vi "vision processing.vi"(6 "Image In":T1, 7 "error in (no error)":errorcluster) -> (11 "error out":errorcluster, 14 "x":dbl, 15 "y":dbl, 16 "left":dbl, 17 "top":dbl, 18 "right":dbl, 19 "bottom":dbl)   [LabVIEW 2012]
uses:
  <vilib>/vision/Image Controls.llb/IMAQ Image.ctl
  typedefs/fg_typedef.ctl
  <vilib>/vision/NI_Vision_Development_Module.lvlib
panel:
  out "Cam":T1(plugin-control)
  out "# Particles":i32
  in  "error in":errorcluster
  out "Image Out":T1
  out "error out":errorcluster
  out "Number of Particles Found":i32
  out "Image Out":T1(plugin-control)
  out "Number of Targets Found":i32
  # "0  center of mass x\n1  center of mass y\n2  first pixel x\n3  first pixel y\n4  bounding rect left\n5  bounding rect top\n6  bounding rect right\n7  bounding rect bottom\n8 max feret diameter start x\n9  max feret diameter start y\n10 max feret diameter end x\n11 max feret diameter end y\n12 max horiz segment length left\n13 max horiz segment length right\n14 max horiz segment length row\n15 bounding rect width \n16 bounding rect height\n17 bounding rect diagional\n..\n33 area"
  # "13'3\"\n3'9\""
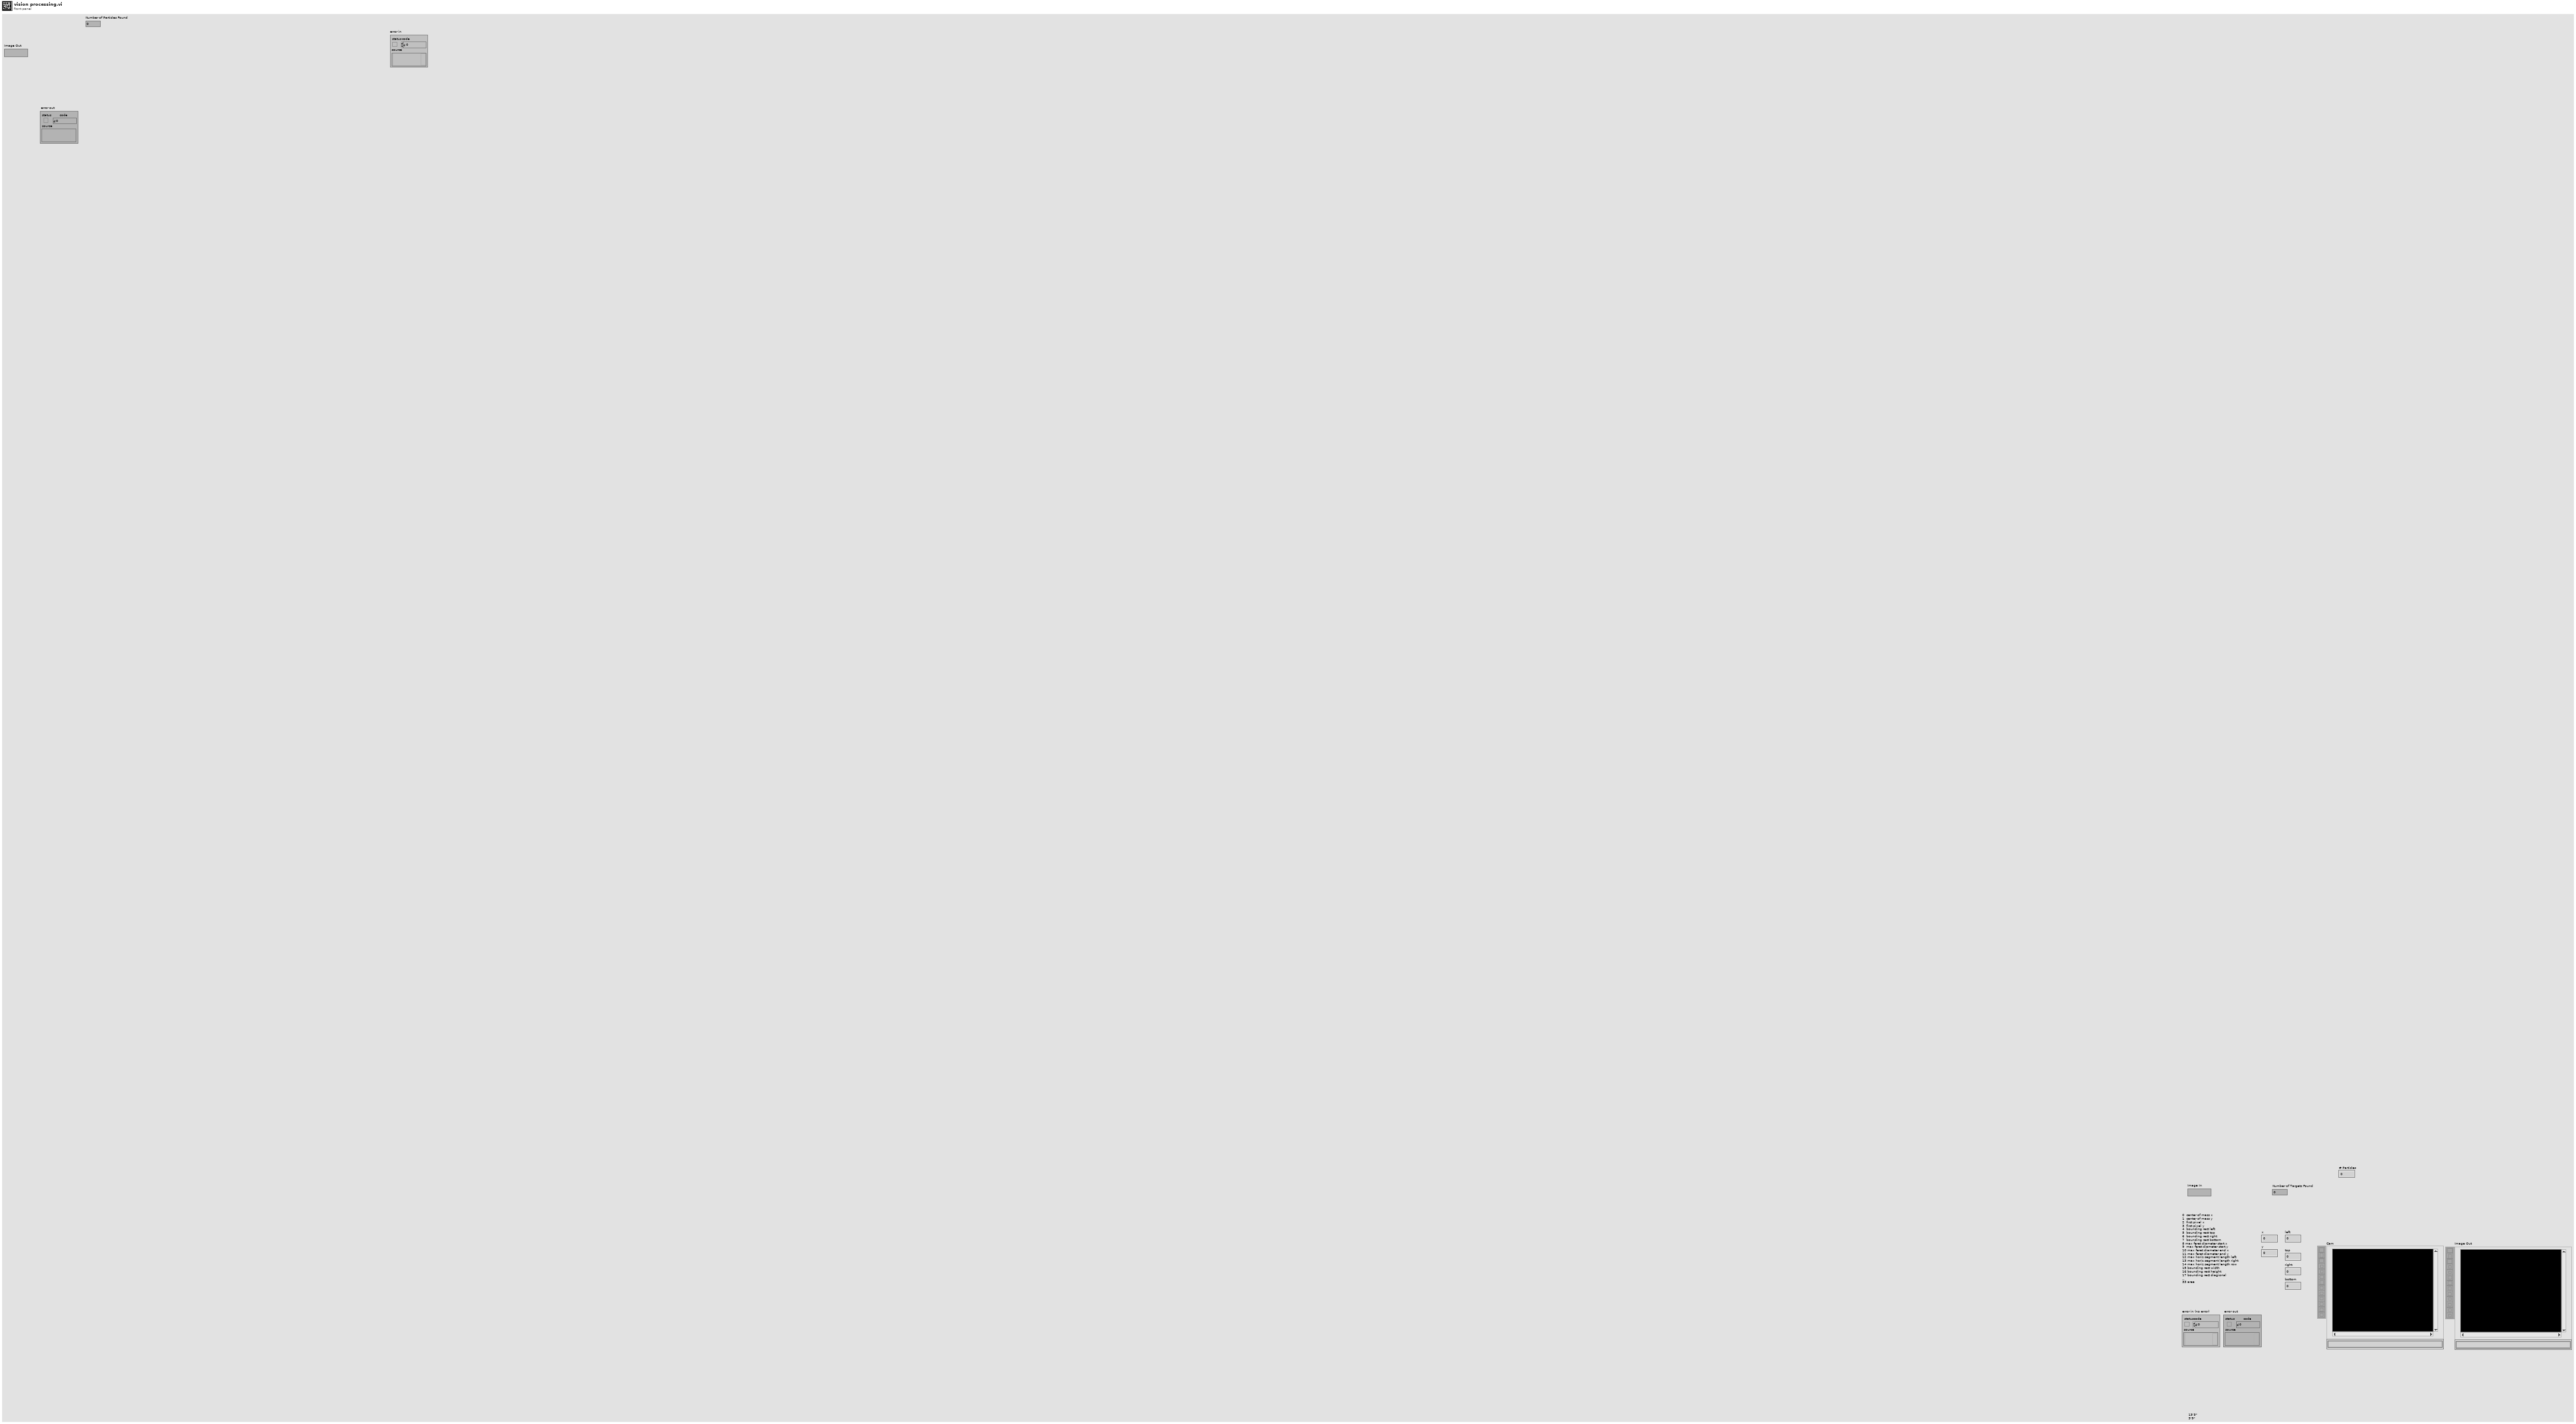
[diagram p1: front panel]
types:
  T1 = typedef "IMAQ Image.ctl" = refnum<image>
  T2 = typedef "Image Type" = u32
  T3 = typedef "fg_typedef.ctl" = enum16{"Get", "Set"}
  T4 = enum32{"AutoM", "Close", "Dilate", "Erode", "Gradient", "Gradient out", "Gradient in", "Hit miss", "Open", "PClose", "POpen", "Thick", "Thin"}
  T5 = cluster{"Brightness":sgl, "Contrast":sgl, "Gamma":sgl}
  T6 = cluster{"Measurement Parameter":i32, "Range Lower Value":dbl, "Range Upper Value":dbl, "Range":bool, "Measurement Type":bool}[]
  T7 = typedef "Particle Parameters" = i32
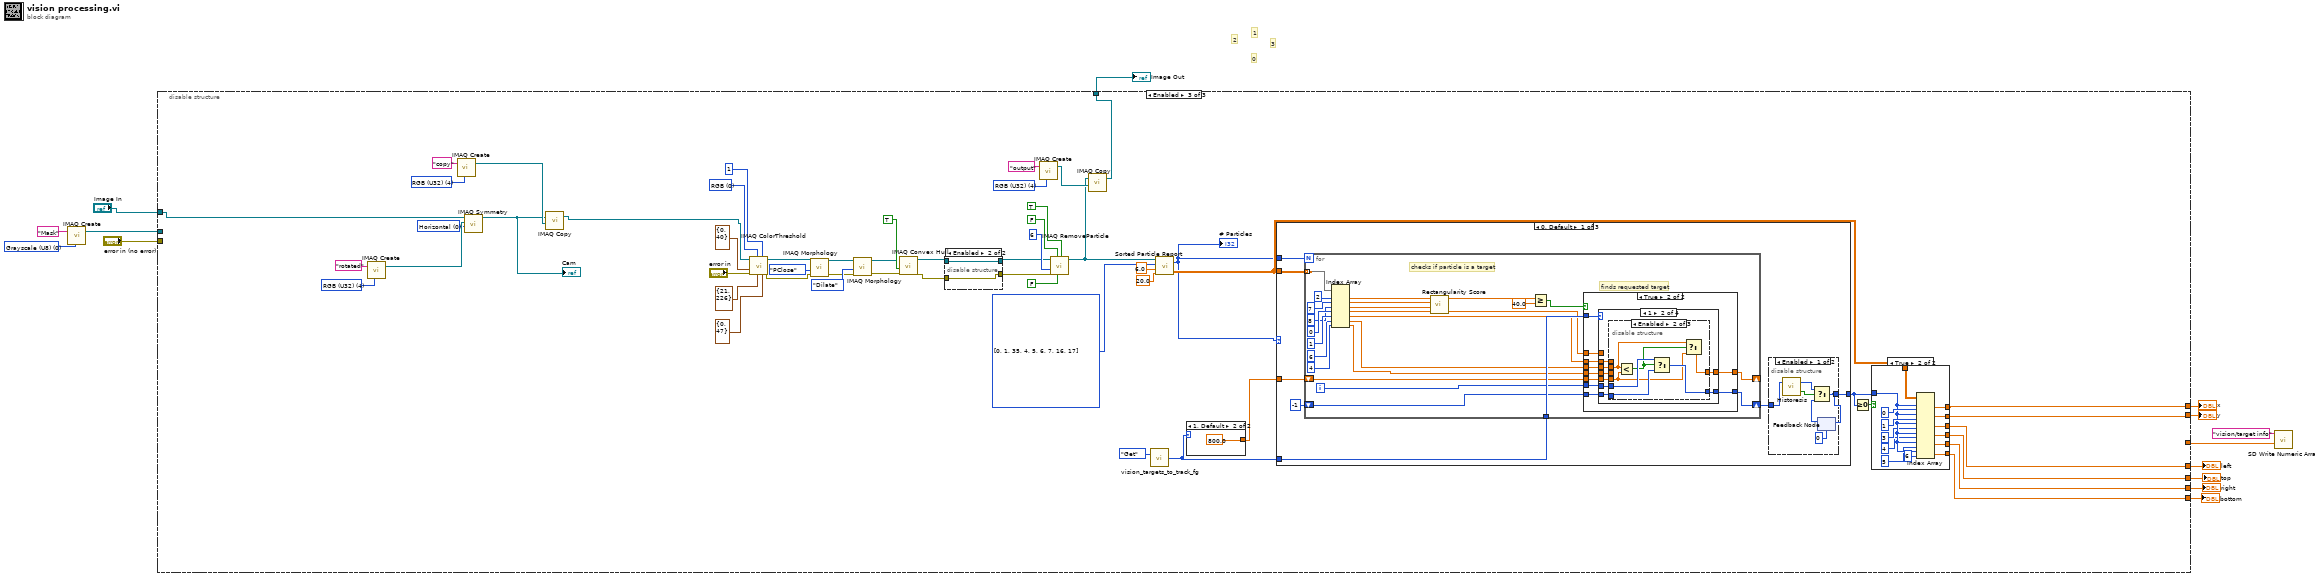
[diagram p0: block diagram]
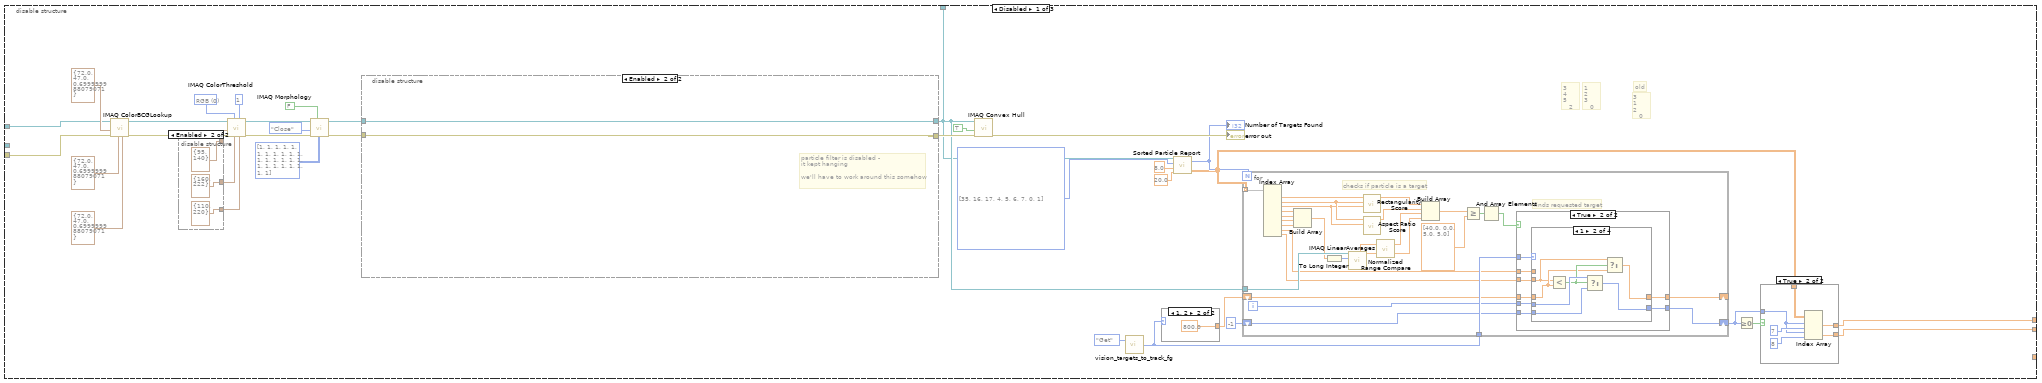
[diagram p2: hidden frame]
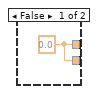
[diagram p3: hidden frame]
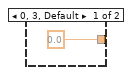
[diagram p4: hidden frame]
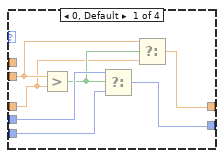
[diagram p6: hidden frame]
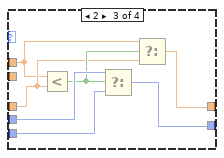
[diagram p7: hidden frame]
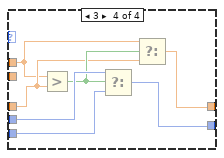
[diagram p8: hidden frame]
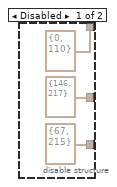
[diagram p9: hidden frame]
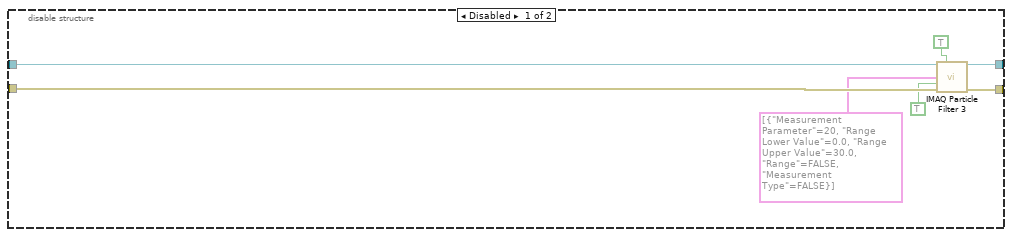
[diagram p10: hidden frame]
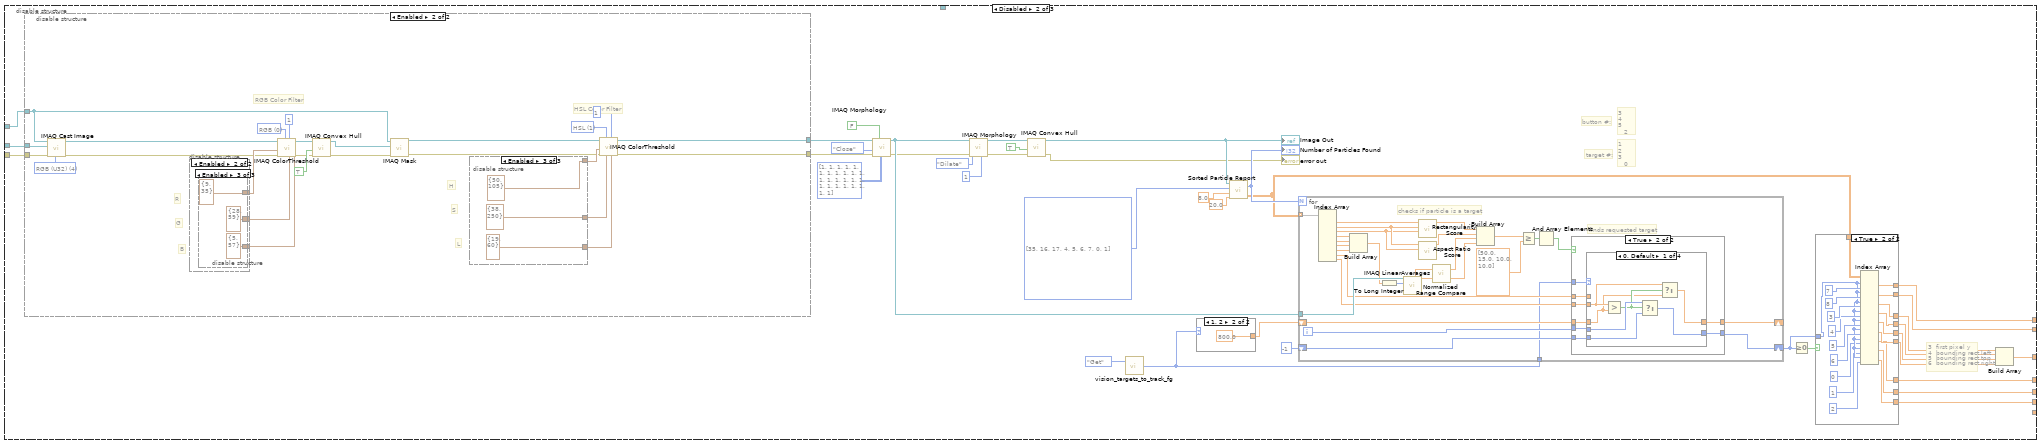
[diagram p11: hidden frame]
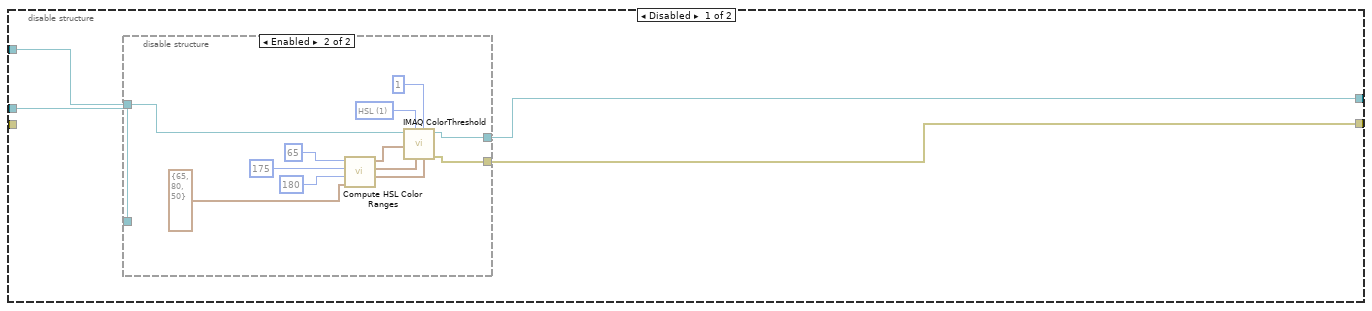
[diagram p12: hidden frame]
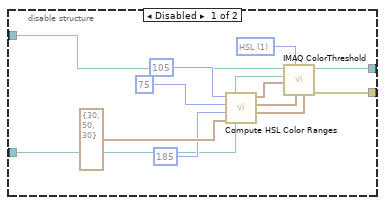
[diagram p13: hidden frame]
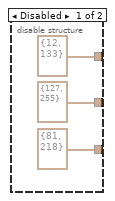
[diagram p14: hidden frame]
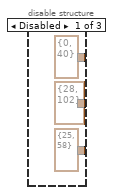
[diagram p15: hidden frame]
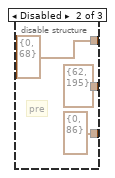
[diagram p16: hidden frame]
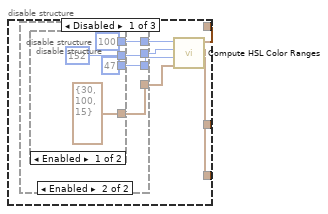
[diagram p17: hidden frame]
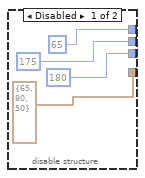
[diagram p18: hidden frame]
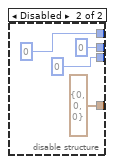
[diagram p19: hidden frame]
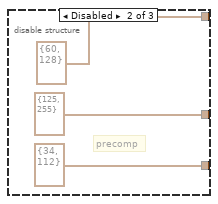
[diagram p20: hidden frame]
diagram:
  w11 = T2 0 items=["Grayscale (U8)", "Grayscale (I16)", "Grayscale (SGL)", "Complex (CSG)", "RGB (U32)", "HSL (U32)", "RGB (U64)", "Grayscale (U16)"] ("Image Type")
  # "3"
  # "2"
  # "1"
  # "0"
  n1 = call "IMAQ Create"("Image Name"="Mask", "Image Type"=w11) -> ("New Image"=w10:T1)  [unwired: 2 in, 2 out]
  n2 = disable-structure shown="Enabled" {
    disable-tunnel: "error in (no error)" -> [w32 w154 _]
    disable-tunnel: "Image In" -> [w31 w166 w372]
    disable-tunnel: [w17 w163 w384] -> w9
    disable-tunnel: [w16 w144 w373] -> w8
    disable-tunnel: w10 -> [_ w155 _]
    disable-tunnel: [_ w153 w383] -> w7
    disable-tunnel: [_ w152 w374] -> w6
    disable-tunnel: [_ w151 w382] -> w5
    disable-tunnel: [_ w143 _] -> w4
    disable-tunnel: [w15 _ w391] -> w2
    disable-tunnel: [_ _ w375] -> w1
    frame Disabled {
      w24 = T7[] [35, 16, 17, 4, 5, 6, 7, 0, 1] items=["Center of Mass X", "Center of Mass Y", "First Pixel X", "First Pixel Y", "Bounding Rect Left", "Bounding Rect Top", "Bounding Rect Right", "Bounding Rect Bottom", "Max Feret Diameter Start X", "Max Feret Diameter Start Y", "Max Feret Diameter End X", "Max Feret Diameter End Y", "Max Horiz. Segment Length Left", "Max Horiz. Segment Length Right", "Max Horiz. Segment Length Row", "-", "Bounding Rect Width", "Bounding Rect Height", "Bounding Rect Diagonal", "Perimeter", "Convex Hull Perimeter", "Holes' Perimeter", "Max Feret Diameter", "Equivalent Ellipse Major Axis", "Equivalent Ellipse Minor Axis", "Equivalent Ellipse Minor Axis (Feret)", "Equivalent Rect Long Side", "Equivalent Rect Short Side", "Equivalent Rect Diagonal", "Equivalent Rect Short Side (Feret)", "Average Horiz. Segment Length", "Average Vert. Segment Length", "Hydraulic Radius", "Waddel Disk Diameter", "-", "Area", "Holes' Area", "Particle & Holes' Area", "Convex Hull Area", "Image Area", "-", "Number of Holes", "Number of Horiz. Segments", "Number of Vert. Segments", "-", "Orientation", "Max Feret Diameter Orientation", "-", "% Area/Image Area", "% Area/(Particle & Holes' Area)", "Ratio of Equivalent Ellipse Axes", "Ratio of Equivalent Rect Sides", "-", "Elongation Factor", "Compactness Factor", "Heywood Circularity Factor", "Type Factor", "-", "Sum X", "Sum Y", "Sum XX", "Sum XY", "Sum YY", "Sum XXX", "Sum XXY", "Sum XYY", "Sum YYY", "-", "Moment of Inertia XX", "Moment of Inertia XY", "Moment of Inertia YY", "Moment of Inertia XXX", "Moment of Inertia XXY", "Moment of Inertia XYY", "Moment of Inertia YYY", "Norm. Moment of Inertia XX", "Norm. Moment of Inertia XY", "Norm. Moment of Inertia YY", "Norm. Moment of Inertia XXX", "Norm. Moment of Inertia XXY", "Norm. Moment of Inertia XYY", "Norm. Moment of Inertia YYY", "Hu Moment 1", "Hu Moment 2", "Hu Moment 3", "Hu Moment 4", "Hu Moment 5", "Hu Moment 6", "Hu Moment 7"] ("Requested Particle Measurements")
      w46 = u16 0 items=["RGB", "HSL", "HSV", "HSI"] ("Color Mode")
      # "old"
      # "1   \n2     3\n   0"
      # "3   \n1     2\n   0"
      # "3   \n4     5\n   2"
      n3 = call "IMAQ ColorBCGLookup"("Blue BCG Values"=T5 {"Brightness"=72.0, "Contrast"=47.0, "Gamma"=0.7}, "Green BCG Values"=T5 {"Brightness"=72.0, "Contrast"=47.0, "Gamma"=0.7}, "error in (no error)"=w32, "Red BCG Values"=T5 {"Brightness"=72.0, "Contrast"=47.0, "Gamma"=0.7}, "Image Src"=w31) -> ("error out"=w51:errorcluster, "Image Dst Out"=w42:T1)  [unwired: 2 in, 3 out]
      n4 = disable-structure shown="Enabled" {
        disable-tunnel: [cluster{"Lower value":i32, "Upper value":i32} {"Lower value"=0, "Upper value"=110} ("Red or Hue Range") cluster{"Lower value":i32, "Upper value":i32} {"Lower value"=95, "Upper value"=140} ("Red or Hue Range")] -> w45
        disable-tunnel: [cluster{"Lower value":i32, "Upper value":i32} {"Lower value"=146, "Upper value"=217} ("Green or Sat Range") cluster{"Lower value":i32, "Upper value":i32} {"Lower value"=160, "Upper value"=222} ("Green or Sat Range")] -> w44
        disable-tunnel: [cluster{"Lower value":i32, "Upper value":i32} {"Lower value"=67, "Upper value"=215} ("Blue or Luma or Val or Inten Range") cluster{"Lower value":i32, "Upper value":i32} {"Lower value"=110, "Upper value"=220} ("Blue or Luma or Val or Inten Range")] -> w43
        frame Disabled {
        }
        frame Enabled {
        }
      }
      n5 = call "IMAQ ColorThreshold"("Blue or Luma or Val or Inten Range"=w43, "Replace Value"=1, "Green or Sat Range"=w44, "Color Mode"=w46, "error in (no error)"=w51, "Red or Hue Range"=w45, "Image Src"=w42) -> ("error out"=w41:errorcluster, "Image Dst Out"=w37:T1)  [unwired: 1 in, 2 out]
      n6 = call "IMAQ Morphology"("Structuring Element"=i32[][] [[1, 1, 1, 1, 1], [1, 1, 1, 1, 1], [1, 1, 1, 1, 1], [1, 1, 1, 1, 1], [1, 1, 1, 1, 1]], "Square/Hexa (Square)"=FALSE, "error in (no error)"=w41, "Operation"=T4."Close", "Image Src"=w37) -> ("error out"=w36:errorcluster, "Image Dst Out"=w34:T1)  [unwired: 2 in, 3 out]
      n7 = disable-structure shown="Enabled" {
        disable-tunnel: w36 -> [w140 w142]
        disable-tunnel: [w137 w142] -> w35
        disable-tunnel: w34 -> [w136 w141]
        disable-tunnel: [w134 w141] -> w30
        frame Disabled {
          n8 = call "IMAQ Particle Filter 3"("Image Src"=w136, "Connectivity 4/8 (8)"=TRUE, "Selection Values"=T6 [{"Measurement Parameter"=20, "Range Lower Value"=0.0, "Range Upper Value"=30.0, "Range"=FALSE, "Measurement Type"=FALSE}], "Keep/Remove Particles (F)"=TRUE ("Keep/Remove Particles"), "error in (no error)"=w140) -> ("Image Dst Out"=w134:T1, "error out"=w137:errorcluster)  [unwired: 4 in, 5 out]
        }
        frame Enabled {
          # "particle filter is disabled - \nit kept hanging\n\nwe'll have to work around this somehow"
        }
      }
      n9 = call "IMAQ Convex Hull"("error in (no error)"=w35, "Connectivity 4/8 (8)"=TRUE, "Image Src"=w30) -> ("error out"=→"error out":errorcluster, "Image Dst Out"=w15:T1)  [unwired: 1 in, 6 out]
      n10 = call "vision_targets_to_track_fg.vi"("Menu (Get)"=fg_typedef."Get") -> ("Output"=w27:i32)  [unwired: 1 in]
      n11 = case shown="1, 2" w27 {
        tunnel: [0.0 ("element") 800.0 ("element")] -> w28
        frame 0, 3, Default {
        }
        frame 1, 2 {
        }
      }
      n12 = call "Sorted Particle Report.vi"("Area Size Limit"=20.0, "Particle Count Limit"=8.0, "Pixel Measurements"=w24, "Image in"=w15) -> ("Sorted Data"=w20:dbl[][], "Particles"=w21:i32)
      "Number of Targets Found" <- w21
      n13 = for {
        N: w21 -> [_]
        tunnel: w30 -> [w89]
        tunnel: w20 -> [w88] mode=indexing
        tunnel: w27 -> [w78]
        shift-right: [w70] -> _
        shift-left: w28 -> [w73]
        shift-right: [w71] -> w19
        shift-left: -1 -> [w72]
        i -> [w74]
        # "checks if particle is a target"
        # "finds requested target"
        n14 = Index Array(array=w88) -> (element #1=w69:dbl, element #2=w66:dbl, element #3=w65:dbl, element #4=w84:dbl, element #5=w83:dbl, element #6=w82:dbl, element #7=w81:dbl, element #8=w76:dbl, element #9=w77:dbl)  [unwired: 9 in]
        n15 = Build Array(w84, w83, w82, w81) -> (w80:dbl[])
        n16 = To Long Integer(number=w80) -> (32bit integer=w79:i32[])
        n17 = call "IMAQ LinearAverages"("Optional Rectangle"=w79, "Image Src"=w89) -> ("Y Axis Averages"=w61:sgl[], "X Axis Averages"=w62:sgl[])  [unwired: 2 in, 6 out]
        n18 = call "Rectangularity Score.vi"("Height"=w65, "Width"=w66, "Area"=w69) -> ("Score"=w68:dbl)  [unwired: 8 in]
        n19 = call "Aspect Ratio Score.vi"("Height"=w65, "Width"=w66) -> ("Score"=w67:dbl)  [unwired: 9 in]
        n20 = call "Normalized Range Compare.vi"("Y Averages"=w61, "X Averages"=w62) -> ("Y Score"=w63:dbl, "X Score"=w64:dbl)
        n21 = Build Array(w68, w67, w64, w63) -> (w87:dbl[])
        n22 = Greater Or Equal?(x=w87, y=dbl[] [40.0, 0.0, 5.0, 5.0]) -> (x >= y?=w85:bool[])
        n23 = And Array Elements(Boolean array=w85) -> (logical AND=w75:bool)
        n24 = case shown="True" w75 {
          tunnel: w78 -> [_ w99]
          tunnel: w77 -> [_ w98]
          tunnel: w76 -> [_ w97]
          tunnel: w74 -> [_ w96]
          tunnel: w73 -> [w90 w95]
          tunnel: w72 -> [w91 w94]
          tunnel: [w91 w93] -> w71
          tunnel: [w90 w92] -> w70
          frame False {
          }
          frame True {
            n25 = case shown="1" w99 {
              tunnel: w98 -> [w102 w107 _ _]
              tunnel: w97 -> [_ _ w114 w121]
              tunnel: w96 -> [w106 w113 w120 w127]
              tunnel: w95 -> [w101 w109 w116 w123]
              tunnel: w94 -> [w105 w112 w119 w126]
              tunnel: [w104 w111 w118 w125] -> w93
              tunnel: [w100 w108 w115 w122] -> w92
              frame 0, Default {
                n26 = Greater?(x=w102, y=w101) -> (0:w103:bool)
                n27 = Select(t=w106, s=w103, f=w105) -> (s? t:f=w104:i32)
                n28 = Select(t=w102, s=w103, f=w101) -> (s? t:f=w100:dbl)
              }
              frame 1 {
                n29 = Less?(x=w107, y=w109) -> (x < y?=w110:bool)
                n30 = Select(t=w113, s=w110, f=w112) -> (s? t:f=w111:i32)
                n31 = Select(t=w107, s=w110, f=w109) -> (s? t:f=w108:dbl)
              }
              frame 2 {
                n32 = Less?(x=w114, y=w116) -> (x < y?=w117:bool)
                n33 = Select(t=w120, s=w117, f=w119) -> (s? t:f=w118:i32)
                n34 = Select(t=w114, s=w117, f=w116) -> (s? t:f=w115:dbl)
              }
              frame 3 {
                n35 = Greater?(x=w121, y=w123) -> (0:w124:bool)
                n36 = Select(t=w127, s=w124, f=w126) -> (s? t:f=w125:i32)
                n37 = Select(t=w121, s=w124, f=w123) -> (s? t:f=w122:dbl)
              }
            }
          }
        }
      }
      n38 = Greater Or Equal To 0?(x=w19) -> (x >= 0?=w18:bool)
      n39 = case shown="True" w18 {
        tunnel: [w52 w56] -> w17
        tunnel: [w52 w55] -> w16
        tunnel: w20 -> [_ w54]
        tunnel: w19 -> [_ w53]
        frame False {
          w52 = 0.0 ("Numeric")
        }
        frame True {
          n40 = Index Array(array=w54, index (row) #1=w53, index (col) #1=7, index (row) #2=w53, index (col) #2=8) -> (element #1=w56:dbl, element #2=w55:dbl)
        }
      }
    }
    frame Disabled {
      w165 = T7[] [35, 16, 17, 4, 5, 6, 7, 0, 1] items=["Center of Mass X", "Center of Mass Y", "First Pixel X", "First Pixel Y", "Bounding Rect Left", "Bounding Rect Top", "Bounding Rect Right", "Bounding Rect Bottom", "Max Feret Diameter Start X", "Max Feret Diameter Start Y", "Max Feret Diameter End X", "Max Feret Diameter End Y", "Max Horiz. Segment Length Left", "Max Horiz. Segment Length Right", "Max Horiz. Segment Length Row", "-", "Bounding Rect Width", "Bounding Rect Height", "Bounding Rect Diagonal", "Perimeter", "Convex Hull Perimeter", "Holes' Perimeter", "Max Feret Diameter", "Equivalent Ellipse Major Axis", "Equivalent Ellipse Minor Axis", "Equivalent Ellipse Minor Axis (Feret)", "Equivalent Rect Long Side", "Equivalent Rect Short Side", "Equivalent Rect Diagonal", "Equivalent Rect Short Side (Feret)", "Average Horiz. Segment Length", "Average Vert. Segment Length", "Hydraulic Radius", "Waddel Disk Diameter", "-", "Area", "Holes' Area", "Particle & Holes' Area", "Convex Hull Area", "Image Area", "-", "Number of Holes", "Number of Horiz. Segments", "Number of Vert. Segments", "-", "Orientation", "Max Feret Diameter Orientation", "-", "% Area/Image Area", "% Area/(Particle & Holes' Area)", "Ratio of Equivalent Ellipse Axes", "Ratio of Equivalent Rect Sides", "-", "Elongation Factor", "Compactness Factor", "Heywood Circularity Factor", "Type Factor", "-", "Sum X", "Sum Y", "Sum XX", "Sum XY", "Sum YY", "Sum XXX", "Sum XXY", "Sum XYY", "Sum YYY", "-", "Moment of Inertia XX", "Moment of Inertia XY", "Moment of Inertia YY", "Moment of Inertia XXX", "Moment of Inertia XXY", "Moment of Inertia XYY", "Moment of Inertia YYY", "Norm. Moment of Inertia XX", "Norm. Moment of Inertia XY", "Norm. Moment of Inertia YY", "Norm. Moment of Inertia XXX", "Norm. Moment of Inertia XXY", "Norm. Moment of Inertia XYY", "Norm. Moment of Inertia YYY", "Hu Moment 1", "Hu Moment 2", "Hu Moment 3", "Hu Moment 4", "Hu Moment 5", "Hu Moment 6", "Hu Moment 7"] ("Requested Particle Measurements")
      # "3  first pixel y\n4  bounding rect left\n5  bounding rect top\n6  bounding rect right"
      # "target #:"
      # "button #:"
      # "1   \n2     3\n   0"
      # "3   \n4     5\n   2"
      n41 = disable-structure shown="Enabled" {
        disable-tunnel: [w184 w223] -> w177
        disable-tunnel: [w183 w224] -> w176
        disable-tunnel: w166 -> [w182 w209]
        disable-tunnel: w155 -> [w181 w233]
        disable-tunnel: w154 -> [_ w232]
        frame Disabled {
          n42 = disable-structure shown="Enabled" {
            disable-tunnel: [w196 w199] -> w184
            disable-tunnel: [w195 w200] -> w183
            disable-tunnel: w182 -> [w186 w198]
            disable-tunnel: w181 -> [w185 _]
            frame Disabled {
              w194 = u16 1 items=["RGB", "HSL", "HSV", "HSI"] ("Color Mode")
              n43 = call "Compute HSL Color Ranges.vi"("Margins"=cluster{"Hue":i32, "Sat":i32, "Lum":i32} {"Hue"=30, "Sat"=50, "Lum"=30}, "Luminance"=185, "Saturation"=75, "Hue"=105) -> ("Lum Range"=w191:cluster{i32, i32}, "Sat Range"=w192:cluster{i32, i32}, "Hue Range"=w193:cluster{i32, i32})  [unwired: 5 in]
              n44 = call "IMAQ ColorThreshold"("Blue or Luma or Val or Inten Range"=w191, "Green or Sat Range"=w192, "Color Mode"=w194, "Red or Hue Range"=w193, "Image Dst"=w185, "Image Src"=w186) -> ("error out"=w196:errorcluster, "Image Dst Out"=w195:T1)  [unwired: 4 in]
            }
            frame Enabled {
              w202 = u16 1 items=["RGB", "HSL", "HSV", "HSI"] ("Color Mode")
              n45 = call "Compute HSL Color Ranges.vi"("Margins"=cluster{"Hue":i32, "Sat":i32, "Lum":i32} {"Hue"=65, "Sat"=80, "Lum"=50}, "Luminance"=180, "Saturation"=175, "Hue"=65) -> ("Lum Range"=w205:cluster{i32, i32}, "Sat Range"=w204:cluster{i32, i32}, "Hue Range"=w203:cluster{i32, i32})  [unwired: 5 in]
              n46 = call "IMAQ ColorThreshold"("Blue or Luma or Val or Inten Range"=w205, "Replace Value"=1, "Green or Sat Range"=w204, "Color Mode"=w202, "Red or Hue Range"=w203, "Image Src"=w198) -> ("error out"=w199:errorcluster, "Image Dst Out"=w200:T1)  [unwired: 4 in]
            }
          }
        }
        frame Enabled {
          w220 = u16 0 items=["RGB", "HSL", "HSV", "HSI"] ("Color Mode")
          w222 = T2 4 items=["Grayscale (U8)", "Grayscale (I16)", "Grayscale (SGL)", "Complex (CSG)", "RGB (U32)", "HSL (U32)", "RGB (U64)"] ("Image Type")
          w228 = u16 1 items=["RGB", "HSL", "HSV", "HSI"] ("Color Mode")
          # "L"
          # "S"
          # "H"
          # "B"
          # "G"
          # "R"
          # "HSL Color Filter"
          # "RGB Color Filter"
          n47 = call "IMAQ Cast Image"("Image Type"=w222, "error in (no error)"=w232, "Image Dst"=w233, "Image Src"=w209) -> ("error out"=w211:errorcluster, "Image Dst Out"=w218:T1)  [unwired: 6 in]
          n48 = disable-structure shown="Enabled" {
            disable-tunnel: [cluster{"Lower value":i32, "Upper value":i32} {"Lower value"=12, "Upper value"=133} ("Red or Hue Range") w239] -> w214
            disable-tunnel: [cluster{"Lower value":i32, "Upper value":i32} {"Lower value"=127, "Upper value"=255} ("Green or Sat Range") w238] -> w213
            disable-tunnel: [cluster{"Lower value":i32, "Upper value":i32} {"Lower value"=81, "Upper value"=218} ("Blue or Luma or Val or Inten Range") w237] -> w210
            frame Disabled {
            }
            frame Enabled {
              n49 = disable-structure shown="Enabled" {
                disable-tunnel: [cluster{"Lower value":i32, "Upper value":i32} {"Lower value"=0, "Upper value"=40} ("Red or Hue Range") cluster{"Lower value":i32, "Upper value":i32} {"Lower value"=0, "Upper value"=68} ("Red or Hue Range") cluster{"Lower value":i32, "Upper value":i32} {"Lower value"=9, "Upper value"=35} ("Red or Hue Range")] -> w239
                disable-tunnel: [cluster{"Lower value":i32, "Upper value":i32} {"Lower value"=28, "Upper value"=102} ("Green or Sat Range") cluster{"Lower value":i32, "Upper value":i32} {"Lower value"=62, "Upper value"=195} ("Green or Sat Range") cluster{"Lower value":i32, "Upper value":i32} {"Lower value"=28, "Upper value"=59} ("Green or Sat Range")] -> w238
                disable-tunnel: [cluster{"Lower value":i32, "Upper value":i32} {"Lower value"=25, "Upper value"=58} ("Blue or Luma or Val or Inten Range") cluster{"Lower value":i32, "Upper value":i32} {"Lower value"=0, "Upper value"=86} ("Blue or Luma or Val or Inten Range") cluster{"Lower value":i32, "Upper value":i32} {"Lower value"=5, "Upper value"=57} ("Blue or Luma or Val or Inten Range")] -> w237
                frame Disabled {
                }
                frame Disabled {
                  # "pre"
                }
                frame Enabled {
                }
              }
            }
          }
          n50 = call "IMAQ ColorThreshold"("Blue or Luma or Val or Inten Range"=w210, "Replace Value"=1, "Green or Sat Range"=w213, "Color Mode"=w220, "error in (no error)"=w211, "Red or Hue Range"=w214, "Image Src"=w218) -> ("error out"=w216:errorcluster, "Image Dst Out"=w217:T1)  [unwired: 1 in, 2 out]
          n51 = call "IMAQ Convex Hull"("error in (no error)"=w216, "Connectivity 4/8 (8)"=TRUE, "Image Src"=w217) -> ("error out"=w212:errorcluster, "Image Dst Out"=w215:T1)  [unwired: 7 in]
          n52 = call "IMAQ Mask"("error in (no error)"=w212, "Image Mask"=w215, "Image Src"=w209) -> ("error out"=w225:errorcluster, "Image Dst Out"=w226:T1)  [unwired: 2 in]
          n53 = disable-structure shown="Enabled" {
            disable-tunnel: [w251 cluster{"Lower value":i32, "Upper value":i32} {"Lower value"=34, "Upper value"=112} ("Blue or Luma or Val or Inten Range") cluster{"Lower value":i32, "Upper value":i32} {"Lower value"=19, "Upper value"=60} ("Blue or Luma or Val or Inten Range")] -> w231
            disable-tunnel: [w250 cluster{"Lower value":i32, "Upper value":i32} {"Lower value"=125, "Upper value"=255} ("Green or Sat Range") cluster{"Lower value":i32, "Upper value":i32} {"Lower value"=38, "Upper value"=250} ("Green or Sat Range")] -> w230
            disable-tunnel: [w249 cluster{"Lower value":i32, "Upper value":i32} {"Lower value"=60, "Upper value"=128} ("Red or Hue Range") cluster{"Lower value":i32, "Upper value":i32} {"Lower value"=50, "Upper value"=105} ("Red or Hue Range")] -> w229
            frame Disabled {
              n54 = disable-structure shown="Enabled" {
                disable-tunnel: [65 ("Hue") w263] -> w255
                disable-tunnel: [175 ("Saturation") w262] -> w254
                disable-tunnel: [180 ("Luminance") w261] -> w253
                disable-tunnel: [cluster{"Hue":i32, "Sat":i32, "Lum":i32} {"Hue"=65, "Sat"=80, "Lum"=50} ("Margins") w260] -> w252
                frame Disabled {
                }
                frame Enabled {
                  n55 = disable-structure shown="Enabled" {
                    disable-tunnel: [100 ("Hue") 0 ("Hue")] -> w263
                    disable-tunnel: [152 ("Saturation") 0 ("Saturation")] -> w262
                    disable-tunnel: [47 ("Luminance") 0 ("Luminance")] -> w261
                    disable-tunnel: [cluster{"Hue":i32, "Sat":i32, "Lum":i32} {"Hue"=30, "Sat"=100, "Lum"=15} ("Margins") cluster{"Hue":i32, "Sat":i32, "Lum":i32} {"Hue"=0, "Sat"=0, "Lum"=0} ("Margins")] -> w260
                    frame Enabled {
                    }
                    frame Disabled {
                    }
                  }
                }
              }
              n56 = call "Compute HSL Color Ranges.vi"("Margins"=w252, "Luminance"=w253, "Saturation"=w254, "Hue"=w255) -> ("Lum Range"=w251:cluster{i32, i32}, "Sat Range"=w250:cluster{i32, i32}, "Hue Range"=w249:cluster{i32, i32})  [unwired: 5 in]
            }
            frame Disabled {
              # "precomp"
            }
            frame Enabled {
            }
          }
          n57 = call "IMAQ ColorThreshold"("Blue or Luma or Val or Inten Range"=w231, "Replace Value"=1, "Green or Sat Range"=w230, "Color Mode"=w228, "error in (no error)"=w225, "Red or Hue Range"=w229, "Image Src"=w226) -> ("error out"=w223:errorcluster, "Image Dst Out"=w224:T1)  [unwired: 3 in]
        }
      }
      n58 = call "IMAQ Morphology"("Structuring Element"=i32[][] [[1, 1, 1, 1, 1], [1, 1, 1, 1, 1], [1, 1, 1, 1, 1], [1, 1, 1, 1, 1], [1, 1, 1, 1, 1]], "Square/Hexa (Square)"=FALSE, "error in (no error)"=w177, "Operation"=T4."Close", "Image Src"=w176) -> ("error out"=w158:errorcluster, "Image Dst Out"=w160:T1)  [unwired: 2 in, 3 out]
      n59 = call "IMAQ Morphology"("Number of iterations (1)"=1, "error in (no error)"=w158, "Operation"=T4."Dilate", "Image Src"=w160) -> ("error out"=w157:errorcluster, "Image Dst Out"=w159:T1)  [unwired: 6 in]
      n60 = call "IMAQ Convex Hull"("error in (no error)"=w157, "Connectivity 4/8 (8)"=TRUE, "Image Src"=w159) -> ("error out"=→"error out":errorcluster, "Image Dst Out"=w164:T1)  [unwired: 1 in, 6 out]
      "Image Out" <- w164
      n61 = call "vision_targets_to_track_fg.vi"("Menu (Get)"=fg_typedef."Get") -> ("Output"=w149:i32)  [unwired: 1 in]
      n62 = case shown="1, 2" w149 {
        tunnel: [0.0 ("element") 800.0 ("element")] -> w174
        frame 0, 3, Default {
        }
        frame 1, 2 {
        }
      }
      n63 = call "Sorted Particle Report.vi"("Area Size Limit"=20.0, "Particle Count Limit"=8.0, "Pixel Measurements"=w165, "Image in"=w164) -> ("Sorted Data"=w169:dbl[][], "Particles"=w173:i32)
      "Number of Particles Found" <- w173
      n64 = for {
        N: w173 -> [_]
        tunnel: w160 -> [w329]
        tunnel: w169 -> [w328] mode=indexing
        shift-right: [w311] -> _
        shift-left: w174 -> [w314]
        shift-right: [w312] -> w168
        shift-left: -1 -> [w313]
        tunnel: w149 -> [w301]
        i -> [w315]
        # "checks if particle is a target"
        # "finds requested target"
        n65 = Index Array(array=w328) -> (element #1=w310:dbl, element #2=w307:dbl, element #3=w306:dbl, element #4=w324:dbl, element #5=w323:dbl, element #6=w322:dbl, element #7=w321:dbl, element #8=w317:dbl, element #9=w318:dbl)  [unwired: 9 in]
        n66 = Build Array(w324, w323, w322, w321) -> (w320:dbl[])
        n67 = To Long Integer(number=w320) -> (32bit integer=w319:i32[])
        n68 = call "IMAQ LinearAverages"("Optional Rectangle"=w319, "Image Src"=w329) -> ("Y Axis Averages"=w302:sgl[], "X Axis Averages"=w303:sgl[])  [unwired: 2 in, 6 out]
        n69 = call "Rectangularity Score.vi"("Height"=w306, "Width"=w307, "Area"=w310) -> ("Score"=w309:dbl)  [unwired: 8 in]
        n70 = call "Aspect Ratio Score.vi"("Height"=w306, "Width"=w307) -> ("Score"=w308:dbl)  [unwired: 9 in]
        n71 = call "Normalized Range Compare.vi"("Y Averages"=w302, "X Averages"=w303) -> ("Y Score"=w304:dbl, "X Score"=w305:dbl)
        n72 = Build Array(w309, w308, w305, w304) -> (w327:dbl[])
        n73 = Greater Or Equal?(x=w327, y=dbl[] [50.0, 15.0, 10.0, 10.0]) -> (x >= y?=w325:bool[])
        n74 = And Array Elements(Boolean array=w325) -> (logical AND=w316:bool)
        n75 = case shown="True" w316 {
          tunnel: w318 -> [_ w339]
          tunnel: w317 -> [_ w338]
          tunnel: w315 -> [_ w337]
          tunnel: w314 -> [w330 w336]
          tunnel: w313 -> [w331 w335]
          tunnel: [w331 w334] -> w312
          tunnel: [w330 w333] -> w311
          tunnel: w301 -> [_ w332]
          frame False {
          }
          frame True {
            n76 = case shown="0, Default" w332 {
              tunnel: w339 -> [w342 w347 _ _]
              tunnel: w338 -> [_ _ w354 w361]
              tunnel: w337 -> [w346 w353 w360 w367]
              tunnel: w336 -> [w341 w349 w356 w363]
              tunnel: w335 -> [w345 w352 w359 w366]
              tunnel: [w344 w351 w358 w365] -> w334
              tunnel: [w340 w348 w355 w362] -> w333
              frame 0, Default {
                n77 = Greater?(x=w342, y=w341) -> (0:w343:bool)
                n78 = Select(t=w346, s=w343, f=w345) -> (s? t:f=w344:i32)
                n79 = Select(t=w342, s=w343, f=w341) -> (s? t:f=w340:dbl)
              }
              frame 1 {
                n80 = Less?(x=w347, y=w349) -> (x < y?=w350:bool)
                n81 = Select(t=w353, s=w350, f=w352) -> (s? t:f=w351:i32)
                n82 = Select(t=w347, s=w350, f=w349) -> (s? t:f=w348:dbl)
              }
              frame 2 {
                n83 = Less?(x=w354, y=w356) -> (x < y?=w357:bool)
                n84 = Select(t=w360, s=w357, f=w359) -> (s? t:f=w358:i32)
                n85 = Select(t=w354, s=w357, f=w356) -> (s? t:f=w355:dbl)
              }
              frame 3 {
                n86 = Greater?(x=w361, y=w363) -> (0:w364:bool)
                n87 = Select(t=w367, s=w364, f=w366) -> (s? t:f=w365:i32)
                n88 = Select(t=w361, s=w364, f=w363) -> (s? t:f=w362:dbl)
              }
            }
          }
        }
      }
      n89 = Greater Or Equal To 0?(x=w168) -> (x >= 0?=w167:bool)
      n90 = case shown="True" w167 {
        tunnel: [w280 w298] -> w163
        tunnel: [w280 w297] -> w144
        tunnel: w169 -> [_ w296]
        tunnel: w168 -> [_ w287]
        tunnel: [w280 w291] -> w148
        tunnel: [w280 w290] -> w147
        tunnel: [w280 w289] -> w146
        tunnel: [w280 w288] -> w145
        tunnel: [w280 w283] -> w153
        tunnel: [w280 w282] -> w152
        tunnel: [w280 w281] -> w151
        frame False {
          w280 = 0.0 ("Numeric")
        }
        frame True {
          n91 = Index Array(array=w296, index (row) #1=w287, index (col) #1=7, index (row) #2=w287, index (col) #2=8, index (row) #3=w287, index (col) #3=3, index (row) #4=w287, index (col) #4=4, index (row) #5=w287, index (col) #5=5, index (row) #6=w287, index (col) #6=6, index (row) #7=w287, index (col) #7=0, index (row) #8=w287, index (col) #8=1, index (row) #9=w287, index (col) #9=2) -> (element #1=w298:dbl, element #2=w297:dbl, element #3=w291:dbl, element #4=w290:dbl, element #5=w289:dbl, element #6=w288:dbl, element #7=w283:dbl, element #8=w282:dbl, element #9=w281:dbl)
        }
      }
      n92 = Build Array(w148, w147, w146, w145) -> (w143:dbl[])
    }
    frame Enabled {
      w389 = T7[] [0, 1, 35, 4, 5, 6, 7, 16, 17] items=["Center of Mass X", "Center of Mass Y", "First Pixel X", "First Pixel Y", "Bounding Rect Left", "Bounding Rect Top", "Bounding Rect Right", "Bounding Rect Bottom", "Max Feret Diameter Start X", "Max Feret Diameter Start Y", "Max Feret Diameter End X", "Max Feret Diameter End Y", "Max Horiz. Segment Length Left", "Max Horiz. Segment Length Right", "Max Horiz. Segment Length Row", "-", "Bounding Rect Width", "Bounding Rect Height", "Bounding Rect Diagonal", "Perimeter", "Convex Hull Perimeter", "Holes' Perimeter", "Max Feret Diameter", "Equivalent Ellipse Major Axis", "Equivalent Ellipse Minor Axis", "Equivalent Ellipse Minor Axis (Feret)", "Equivalent Rect Long Side", "Equivalent Rect Short Side", "Equivalent Rect Diagonal", "Equivalent Rect Short Side (Feret)", "Average Horiz. Segment Length", "Average Vert. Segment Length", "Hydraulic Radius", "Waddel Disk Diameter", "-", "Area", "Holes' Area", "Particle & Holes' Area", "Convex Hull Area", "Image Area", "-", "Number of Holes", "Number of Horiz. Segments", "Number of Vert. Segments", "-", "Orientation", "Max Feret Diameter Orientation", "-", "% Area/Image Area", "% Area/(Particle & Holes' Area)", "Ratio of Equivalent Ellipse Axes", "Ratio of Equivalent Rect Sides", "-", "Elongation Factor", "Compactness Factor", "Heywood Circularity Factor", "Type Factor", "-", "Sum X", "Sum Y", "Sum XX", "Sum XY", "Sum YY", "Sum XXX", "Sum XXY", "Sum XYY", "Sum YYY", "-", "Moment of Inertia XX", "Moment of Inertia XY", "Moment of Inertia YY", "Moment of Inertia XXX", "Moment of Inertia XXY", "Moment of Inertia XYY", "Moment of Inertia YYY", "Norm. Moment of Inertia XX", "Norm. Moment of Inertia XY", "Norm. Moment of Inertia YY", "Norm. Moment of Inertia XXX", "Norm. Moment of Inertia XXY", "Norm. Moment of Inertia XYY", "Norm. Moment of Inertia YYY", "Hu Moment 1", "Hu Moment 2", "Hu Moment 3", "Hu Moment 4", "Hu Moment 5", "Hu Moment 6", "Hu Moment 7"] ("Requested Particle Measurements")
      w394 = T2 4 items=["Grayscale (U8)", "Grayscale (I16)", "Grayscale (SGL)", "Complex (CSG)", "RGB (U32)", "HSL (U32)", "RGB (U64)", "Grayscale (U16)"] ("Image Type")
      w402 = u32 0 items=["Horizontal", "Vertical", "Central", "1st Diagonal", "2nd Diagonal"] ("Type of Symmetry")
      w405 = T2 4 items=["Grayscale (U8)", "Grayscale (I16)", "Grayscale (SGL)", "Complex (CSG)", "RGB (U32)", "HSL (U32)", "RGB (U64)", "Grayscale (U16)"] ("Image Type")
      w407 = T2 4 items=["Grayscale (U8)", "Grayscale (I16)", "Grayscale (SGL)", "Complex (CSG)", "RGB (U32)", "HSL (U32)", "RGB (U64)", "Grayscale (U16)"] ("Image Type")
      w420 = u16 0 items=["RGB", "HSL", "HSV", "HSI"] ("Color Mode")
      n93 = call "IMAQ Create"("Image Name"="rotated", "Image Type"=w405) -> ("New Image"=w403:T1)  [unwired: 3 in, 1 out]
      n94 = call "IMAQ Create"("Image Name"="copy", "Image Type"=w407) -> ("New Image"=w406:T1)  [unwired: 3 in, 1 out]
      n95 = call "IMAQ Symmetry"("Type of Symmetry"=w402, "Image Dst"=w403, "Image Src"=w372) -> ("Image Dst Out"=w370:T1)  [unwired: 2 in, 1 out]
      "Cam" <- w370
      n96 = call "IMAQ Copy"("Image Dst"=w406, "Image Src"=w370) -> ("Image Dst Out"=w371:T1)  [unwired: 4 in, 1 out]
      n97 = call "IMAQ ColorThreshold"("Blue or Luma or Val or Inten Range"=cluster{"Lower value":i32, "Upper value":i32} {"Lower value"=0, "Upper value"=47}, "Replace Value"=1, "Green or Sat Range"=cluster{"Lower value":i32, "Upper value":i32} {"Lower value"=21, "Upper value"=226}, "Color Mode"=w420, "error in (no error)"="error in", "Red or Hue Range"=cluster{"Lower value":i32, "Upper value":i32} {"Lower value"=0, "Upper value"=40}, "Image Src"=w371) -> ("error out"=w399:errorcluster, "Image Dst Out"=w400:T1)  [unwired: 1 in, 2 out]
      n98 = call "IMAQ Morphology"("error in (no error)"=w399, "Operation"=T4."PClose", "Image Src"=w400) -> ("error out"=w380:errorcluster, "Image Dst Out"=w379:T1)  [unwired: 7 in]
      n99 = call "IMAQ Morphology"("error in (no error)"=w380, "Operation"=T4."Dilate", "Image Src"=w379) -> ("error out"=w377:errorcluster, "Image Dst Out"=w378:T1)  [unwired: 7 in]
      n100 = call "IMAQ Convex Hull"("error in (no error)"=w377, "Connectivity 4/8 (8)"=TRUE, "Image Src"=w378) -> ("error out"=w397:errorcluster, "Image Dst Out"=w398:T1)  [unwired: 1 in, 6 out]
      n101 = disable-structure shown="Enabled" {
        disable-tunnel: w398 -> [w546 w549]
        disable-tunnel: w397 -> [w545 w548]
        disable-tunnel: [w544 w548] -> w396
        disable-tunnel: [w543 w549] -> w395
        frame Disabled {
          n102 = call "IMAQ Morphology"("error in (no error)"=w545, "Operation"=T4."Erode", "Image Src"=w546) -> ("error out"=w544:errorcluster, "Image Dst Out"=w543:T1)  [unwired: 7 in]
        }
        frame Enabled {
        }
      }
      n103 = call "IMAQ Create"("Image Name"="output", "Image Type"=w394) -> ("New Image"=w392:T1)  [unwired: 3 in, 1 out]
      n104 = call "IMAQ RemoveParticle"("Connectivity 4/8 (8)"=TRUE, "Low Pass/High Pass (Low)"=FALSE, "Square/Hexa (Square)"=FALSE, "error in (no error)"=w396, "Number of Erosion"=6, "Image Src"=w395) -> ("Image Dst Out"=w387:T1)  [unwired: 1 in, 4 out]
      n105 = call "IMAQ Copy"("Image Dst"=w392, "Image Src"=w387) -> ("Image Dst Out"=w391:T1)  [unwired: 4 in, 1 out]
      n106 = call "vision_targets_to_track_fg.vi"("Menu (Get)"=fg_typedef."Get") -> ("Output"=w376:i32)  [unwired: 1 in]
      n107 = call "Sorted Particle Report.vi"("Area Size Limit"=20.0, "Particle Count Limit"=6.0, "Pixel Measurements"=w389, "Image in"=w387) -> ("Sorted Data"=w385:dbl[][], "Particles"=w368:i32)
      "# Particles" <- w368
      n108 = case shown="1, Default" w376 {
        tunnel: [0.0 ("element") 800.0 ("element")] -> w388
        frame 2, 3 {
        }
        frame 1, Default {
        }
      }
      n109 = case shown="0, Default" w368 {
        tunnel: w368 -> [w428 _ _]
        tunnel: w388 -> [w426 _ _]
        tunnel: w385 -> [w425 _ _]
        tunnel: w376 -> [w424 _ _]
        tunnel: [w422 1 ("Output") 2 ("Output")] -> w369
        frame 0, Default {
          n110 = for {
            N: w428 -> [_]
            tunnel: w425 -> [w459] mode=indexing
            tunnel: w424 -> [w458]
            shift-right: [w453] -> _
            shift-left: w426 -> [w456]
            shift-right: [w454] -> w423
            shift-left: -1 -> [w455]
            i -> [w457]
            # "checks if particle is a target"
            # "finds requested target"
            n111 = Index Array(array=w459, index #1=2 ("index"), index #2=7 ("index"), index #3=8 ("index"), index #4=0 ("index"), index #5=1 ("index"), index #6=6 ("index"), index #7=4 ("index")) -> (element #1=w450:dbl, element #2=w444:dbl, element #3=w443:dbl, element #4=w451:dbl, element #5=w452:dbl, element #6=w437:dbl, element #7=w436:dbl)
            n112 = call "Rectangularity Score.vi"("Height"=w443, "Width"=w444, "Area"=w450) -> ("Score"=w442:dbl)  [unwired: 8 in]
            n113 = Greater Or Equal?(x=w442, y=40.0) -> (x >= y?=w440:bool)
            n114 = case shown="True" w440 {
              tunnel: w458 -> [_ w471]
              tunnel: w452 -> [_ w470]
              tunnel: w451 -> [_ w469]
              tunnel: w457 -> [_ w468]
              tunnel: w456 -> [w460 w467]
              tunnel: w455 -> [w461 w466]
              tunnel: [w461 w465] -> w454
              tunnel: [w460 w464] -> w453
              tunnel: w437 -> [_ w463]
              tunnel: w436 -> [_ w462]
              frame False {
              }
              frame True {
                n115 = case shown="1" w471 {
                  tunnel: w470 -> [w474 w481 _ _]
                  tunnel: w469 -> [_ _ w510 w517]
                  tunnel: w468 -> [w478 w486 w516 w523]
                  tunnel: w467 -> [w473 w483 w512 w519]
                  tunnel: w466 -> [w477 w485 w515 w522]
                  tunnel: [w476 w484 w514 w521] -> w465
                  tunnel: [w472 w482 w511 w518] -> w464
                  tunnel: w463 -> [_ w480 _ _]
                  tunnel: w462 -> [_ w479 _ _]
                  frame 0, Default {
                    n116 = Greater?(x=w474, y=w473) -> (0:w475:bool)
                    n117 = Select(t=w478, s=w475, f=w477) -> (s? t:f=w476:i32)
                    n118 = Select(t=w474, s=w475, f=w473) -> (s? t:f=w472:dbl)
                  }
                  frame 1 {
                    n119 = disable-structure shown="Enabled" {
                      disable-tunnel: w486 -> [w493 w500 w506]
                      disable-tunnel: w485 -> [w492 w499 w505]
                      disable-tunnel: [w491 w498 w504] -> w484
                      disable-tunnel: w483 -> [w489 w496 w501]
                      disable-tunnel: [w488 w495 w503] -> w482
                      disable-tunnel: w481 -> [w487 _ _]
                      disable-tunnel: w480 -> [_ w494 w508]
                      disable-tunnel: w479 -> [_ _ w509]
                      frame Disabled {
                        n120 = Less?(x=w487, y=w489) -> (x < y?=w490:bool)
                        n121 = Select(t=w493, s=w490, f=w492) -> (s? t:f=w491:i32)
                        n122 = Select(t=w487, s=w490, f=w489) -> (s? t:f=w488:dbl)
                      }
                      frame Enabled {
                        n123 = Less?(x=w494, y=w496) -> (x < y?=w497:bool)
                        n124 = Select(t=w500, s=w497, f=w499) -> (s? t:f=w498:i32)
                        n125 = Select(t=w494, s=w497, f=w496) -> (s? t:f=w495:dbl)
                      }
                      frame Disabled {
                        n126 = Subtract(x=w508, y=w509) -> (x-y=w502:dbl)
                        n127 = Less?(x=w502, y=w501) -> (x < y?=w507:bool)
                        n128 = Select(t=w502, s=w507, f=w501) -> (s? t:f=w503:dbl)
                        n129 = Select(t=w506, s=w507, f=w505) -> (s? t:f=w504:i32)
                      }
                    }
                  }
                  frame 2 {
                    n130 = Greater?(x=w510, y=w512) -> (0:w513:bool)
                    n131 = Select(t=w516, s=w513, f=w515) -> (s? t:f=w514:i32)
                    n132 = Select(t=w510, s=w513, f=w512) -> (s? t:f=w511:dbl)
                  }
                  frame 3 {
                    n133 = Less?(x=w517, y=w519) -> (x < y?=w520:bool)
                    n134 = Select(t=w523, s=w520, f=w522) -> (s? t:f=w521:i32)
                    n135 = Select(t=w517, s=w520, f=w519) -> (s? t:f=w518:dbl)
                  }
                }
              }
            }
          }
          n136 = disable-structure shown="Enabled" {
            disable-tunnel: w423 -> [w433 w435]
            disable-tunnel: [w429 w435] -> w422
            frame Enabled {
              n137 = call "Historesis.vi"("Input"=w433) -> ("Same?"=w432:bool, "Output"=w431:i32)  [unwired: 1 in]
              n138 = feedback #1(0) -> (w430:i32)
              n139 = Select(t=w431, s=w432, f=w430) -> (s? t:f=w429:i32)
              n140 = feedback-in #1(w429) -> ()
            }
            frame Disabled {
            }
          }
        }
        frame 3 {
        }
        frame 4 {
        }
      }
      n141 = Greater Or Equal To 0?(x=w369) -> (x >= 0?=w386:bool)
      n142 = case shown="True" w386 {
        tunnel: [w526 w538] -> w384
        tunnel: [w526 w537] -> w373
        tunnel: w385 -> [_ w536]
        tunnel: w369 -> [_ w535]
        tunnel: [w526 w530] -> w383
        tunnel: [w526 w529] -> w374
        tunnel: [w526 w528] -> w382
        tunnel: [w526 w527] -> w375
        frame False {
          w526 = 0.0 ("Numeric")
        }
        frame True {
          n143 = Index Array(array=w536, index (row) #1=w535, index (col) #1=0, index (row) #2=w535, index (col) #2=1, index (row) #3=w535, index (col) #3=3 ("disabled index (col)"), index (row) #4=w535, index (col) #4=4 ("disabled index (col)"), index (row) #5=w535, index (col) #5=5 ("disabled index (col)"), index (row) #6=w535, index (col) #6=6 ("disabled index (col)")) -> (element #1=w538:dbl, element #2=w537:dbl, element #3=w530:dbl, element #4=w529:dbl, element #5=w528:dbl, element #6=w527:dbl)
        }
      }
    }
  }
  "x" <- w9
  "y" <- w8
  "left" <- w7
  "top" <- w6
  "right" <- w5
  "Image Out" <- w2
  "bottom" <- w1
  n144 = call <vilib>:"SD Write Numeric Array.vi"("Numeric Array"=w4, "Name"="vision/target info") -> ()  [unwired: 8 in, 2 out]
